vi "Facade.vi"(0 "Data In":T4, 2 "Display State In":T2, 3 "Container State":T3) -> (6 "Data Out":T4, 7 "Display State Out":T2, 8 "Action":T1)   [LabVIEW 2015, in "FM Tone.xctl"]
uses:
  FM Tone.xctl
  Data.ctl
  <vilib>/_xctls/Container State.ctl
  State.ctl
  <vilib>/_xctls/Action.ctl
  <vilib>/_xctls/XControlSupport.lvlib
panel:
  in  "Phase (cycles)":dbl
  in  "Depth (Hz)":dbl
  in  "Rate (Hz)":dbl
  in  "Carrier (kHz)":dbl
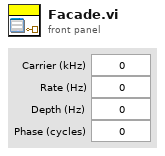
[diagram p1: front panel]
types:
  T1 = typedef "XControlSupport.lvlib/Action.ctl" = cluster{"Data Changed?":bool, "State Changed?":bool, "Action Name":string}
  T2 = typedef "FM Tone.xctl/State.ctl" = cluster{"Numeric":dbl}
  T3 = typedef "XControlSupport.lvlib/Container State.ctl" = cluster{"Indicator?":bool, "Run Mode?":bool, " Refnum":refnum<vi>}
  T4 = typedef "FM Tone.xctl/Data.ctl" = cluster{"Carrier (kHz)":dbl, "ModRate (Hz)":dbl, "Depth (Hz)":dbl, "Phase (cycles)":dbl}
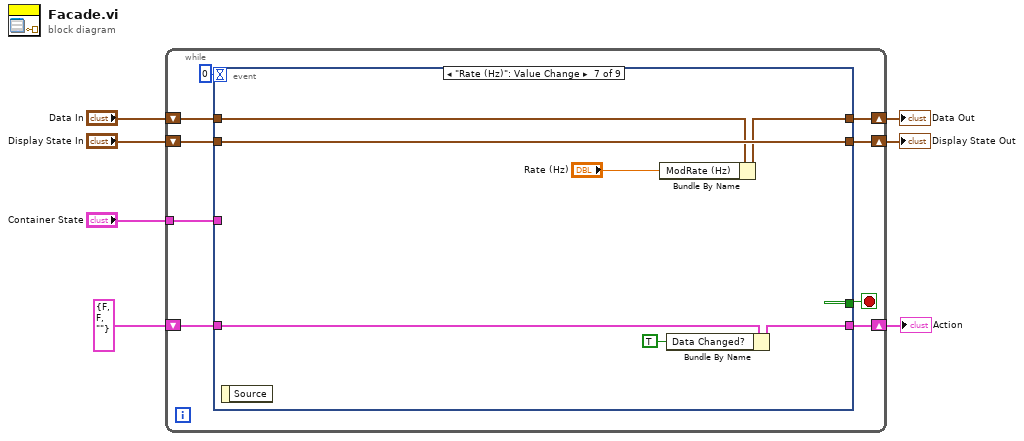
[diagram p0: block diagram]
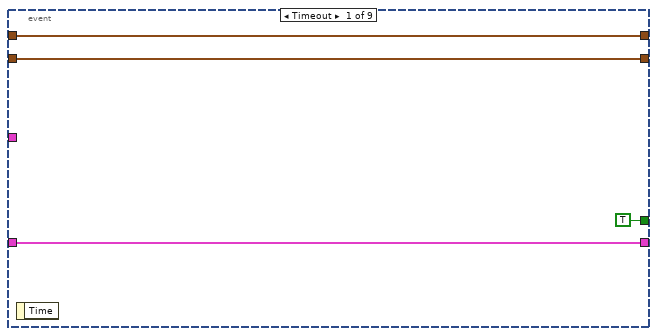
[diagram p2: hidden frame]
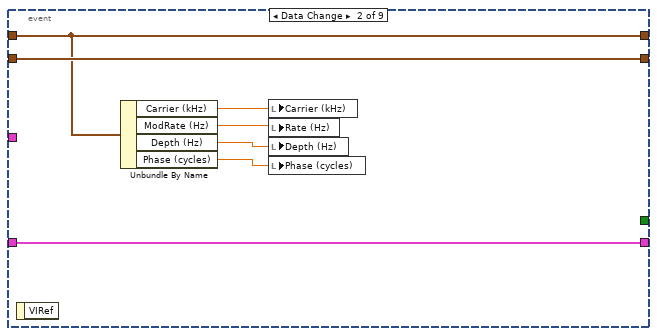
[diagram p3: hidden frame]
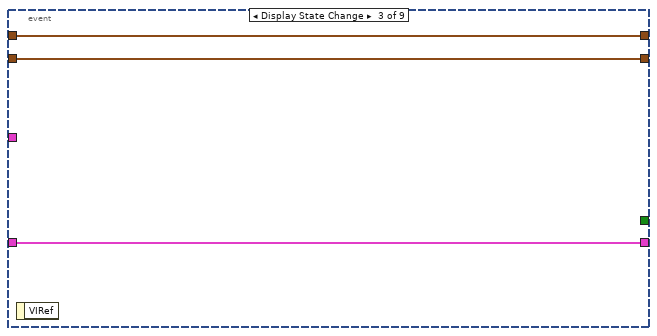
[diagram p4: hidden frame]
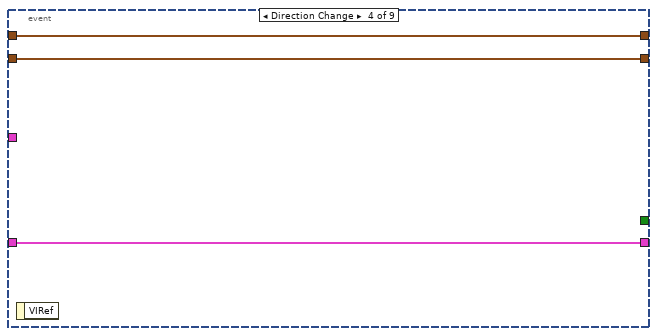
[diagram p5: hidden frame]
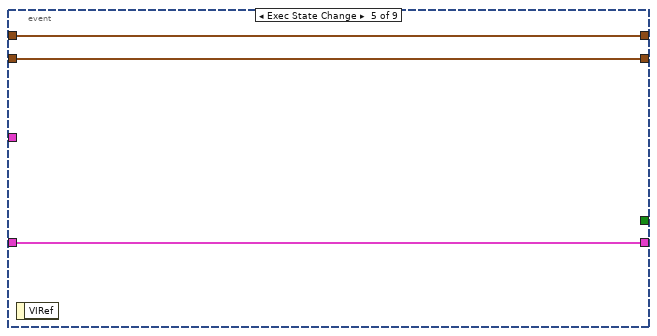
[diagram p6: hidden frame]
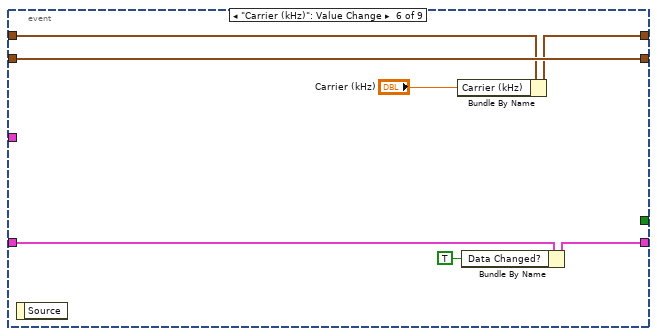
[diagram p7: hidden frame]
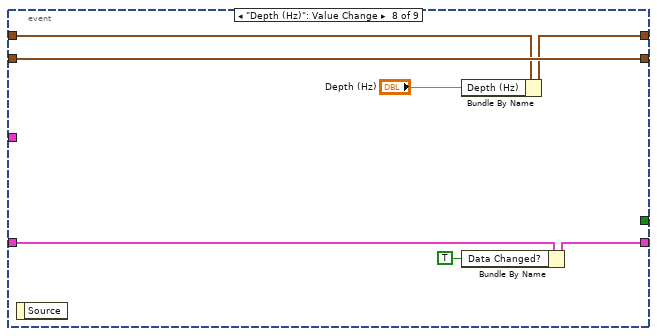
[diagram p8: hidden frame]
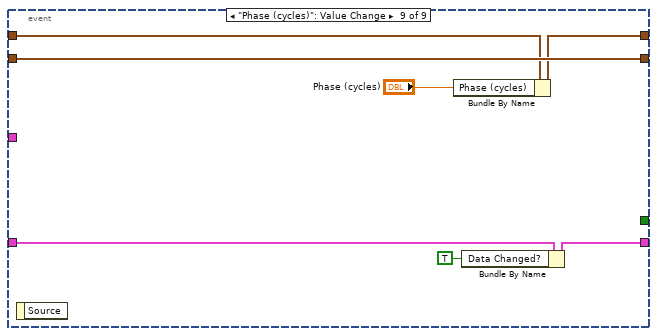
[diagram p9: hidden frame]
diagram:
  n1 = while {
    shift-right: [w15] -> w4
    shift-left: "Display State In" -> [w16]
    tunnel: "Container State" -> [w12]
    shift-right: [w10] -> w7
    shift-left: "Data In" -> [w11]
    shift-right: [w8] -> w2
    shift-left: T1 {"Data Changed?"=FALSE, "State Changed?"=FALSE, "Action Name"=""} ("Action") -> [w9]
    stop <- w14 stop-if-true
    n2 = event shown="[6] \"Rate (Hz)\": Value Change" {
      selector: _ -> [_ _ _ _ _ _ _ _ _]
      dyn-events: _ -> [_ _ _ _ _ _ _ _ _]
      timeout: 0 -> [_ _ _ _ _ _ _ _ _]
      tunnel: w16 -> [w18 w27 w30 w33 w36 w43 w50 w57 w64]
      tunnel: [w18 w27 w30 w33 w36 w43 w50 w57 w64] -> w15
      tunnel: [TRUE _ _ _ _ _ _ _ _] -> w14
      tunnel: w12 -> [_ _ _ _ _ _ _ _ _]
      tunnel: w11 -> [w17 w25 w29 w32 w35 w42 w49 w56 w63]
      tunnel: [w17 w25 w29 w32 w35 w40 w47 w54 w61] -> w10
      tunnel: [w19 w26 w28 w31 w34 w39 w46 w53 w60] -> w8
      tunnel: w9 -> [w19 w26 w28 w31 w34 w41 w48 w55 w62]
      event Timeout {
        n3 = event-data() -> ()  [unwired: 1 in, 1 out]
      }
      event Data Change {
        n4 = event-data() -> ()  [unwired: 1 in, 1 out]
        n5 = Unbundle By Name(w25) -> ("Carrier (kHz)"=w24:dbl, "ModRate (Hz)"=w23:dbl, "Depth (Hz)"=w22:dbl, "Phase (cycles)"=w21:dbl)
        n6 = local write "Carrier (kHz)"(w24) -> ()
        n7 = local write "Rate (Hz)"(w23) -> ()
        n8 = local write "Depth (Hz)"(w22) -> ()
        n9 = local write "Phase (cycles)"(w21) -> ()
      }
      event Display State Change {
        n10 = event-data() -> ()  [unwired: 1 in, 1 out]
      }
      event Direction Change {
        n11 = event-data() -> ()  [unwired: 1 in, 1 out]
      }
      event Exec State Change {
        n12 = event-data() -> ()  [unwired: 1 in, 1 out]
      }
      event "Carrier (kHz)": Value Change {
        n13 = event-data() -> ()  [unwired: 1 in, 1 out]
        n14 = Bundle By Name(cluster=w42, "Carrier (kHz)"="Carrier (kHz)") -> (w40:T4)
        n15 = Bundle By Name(cluster=w41, "Data Changed?"=TRUE) -> (w39:T1)
      }
      event "Rate (Hz)": Value Change {
        n16 = event-data() -> ()  [unwired: 1 in, 1 out]
        n17 = Bundle By Name(cluster=w49, "ModRate (Hz)"="Rate (Hz)") -> (w47:T4)
        n18 = Bundle By Name(cluster=w48, "Data Changed?"=TRUE) -> (w46:T1)
      }
      event "Depth (Hz)": Value Change {
        n19 = event-data() -> ()  [unwired: 1 in, 1 out]
        n20 = Bundle By Name(cluster=w56, "Depth (Hz)"="Depth (Hz)") -> (w54:T4)
        n21 = Bundle By Name(cluster=w55, "Data Changed?"=TRUE) -> (w53:T1)
      }
      event "Phase (cycles)": Value Change {
        n22 = event-data() -> ()  [unwired: 1 in, 1 out]
        n23 = Bundle By Name(cluster=w63, "Phase (cycles)"="Phase (cycles)") -> (w61:T4)
        n24 = Bundle By Name(cluster=w62, "Data Changed?"=TRUE) -> (w60:T1)
      }
    }
  }
  "Display State Out" <- w4
  "Data Out" <- w7
  "Action" <- w2
